vi "Sequence.BuildWaveform.vi"(9 "Rows":cluster{"Start Index":i32, "Length":i32}={"Start Index"=0, "Length"=-1}, 10 "Steps":string[][](array[string]), 11 "Duration":string[](array[string])) -> (1 "Offset":dbl, 2 "Selected":waveform(dbl)[](array[waveform]), 3 "Full":waveform(dbl)[](array[waveform]))   [LabVIEW 2013, in "Simple Sequence Tools - Shared.lvlib"]
uses:
  Simple Sequence Tools - Shared.lvlib
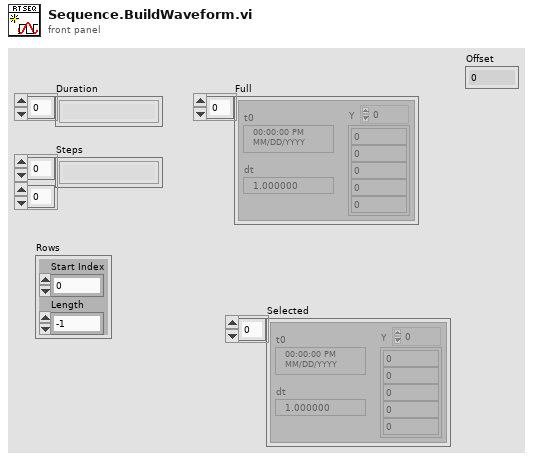
[diagram p1: front panel]
types:
  T1 = typedef "Simple Sequence Tools - Shared.lvlib/Step.Types.ctl" = enum8{"Step", "iStep", "Ramp", "Unchanged", "Unknown", "Sine", "LogSine", "LinearSine", "ForcedRamp", "SquareWave"}
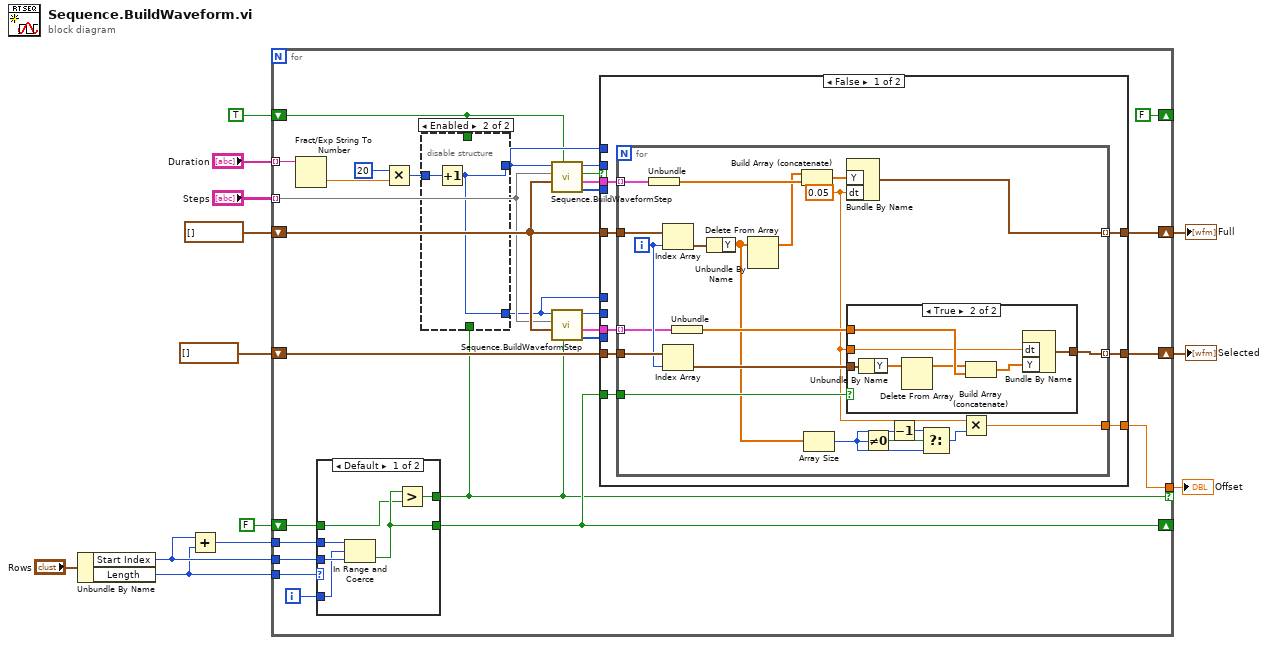
[diagram p0: block diagram]
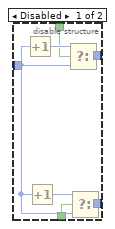
[diagram p2: hidden frame]
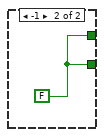
[diagram p3: hidden frame]
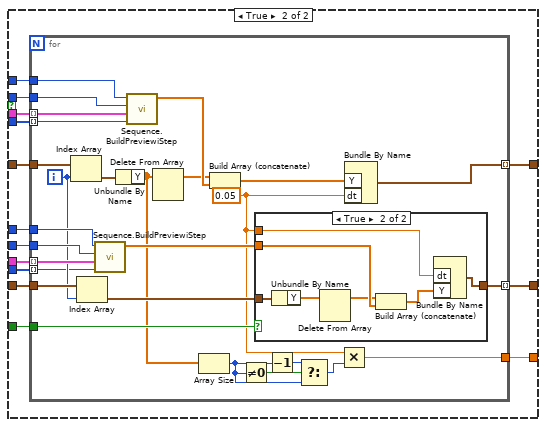
[diagram p5: hidden frame]
diagram:
  n1 = Unbundle By Name("Rows") -> ("Start Index"=w7:i32, "Length"=w6:i32)
  n2 = Add(x=w7, y=w6) -> (x+y=w5:i32)
  n3 = for {
    tunnel: "Steps" -> [w23] mode=indexing
    tunnel: "Duration" -> [w41] mode=indexing
    shift-right: [FALSE] -> _
    shift-left: TRUE -> [w15]
    shift-right: [w34] -> w9
    shift-left: waveform(dbl)[] [] -> [w24]
    tunnel: w6 -> [w33]
    tunnel: w7 -> [w32]
    tunnel: w5 -> [w31]
    shift-right: [w27] -> w3
    shift-left: waveform(dbl)[] [] -> [w28]
    shift-right: [w25] -> _
    shift-left: FALSE -> [w26]
    tunnel: [w18] -> w1 if=w14
    i -> [w30]
    n4 = Fract/Exp String To Number(string=w41) -> (number=w36:dbl)  [unwired: 3 in, 1 out]
    n5 = case shown="Default" w33 {
      tunnel: w32 -> [w56 _]
      tunnel: w31 -> [w55 _]
      tunnel: w30 -> [w54 _]
      tunnel: [w53 w57] -> w25
      tunnel: w26 -> [w52 _]
      tunnel: [w51 w57] -> w14
      frame Default {
        n6 = In Range and Coerce(upper limit=w55, x=w54, lower limit=w56) -> (In Range?=w53:bool)  [unwired: 1 out]
        n7 = Greater?(x=w53, y=w52) -> (0:w51:bool)
      }
      frame -1 {
        w57 = FALSE
      }
    }
    n8 = Multiply(x=u64 20, y=w36) -> (x*y=w22:u64)
    n9 = disable-structure shown="Enabled" {
      disable-tunnel: [w47 w49] -> w35
      disable-tunnel: w22 -> [w45 w50]
      disable-tunnel: [w44 w49] -> w20
      disable-tunnel: w15 -> [w43 _]
      disable-tunnel: w14 -> [w42 _]
      frame Disabled {
        n10 = Increment(x=w45) -> (x+1=w48:u64)
        n11 = Increment(x=w45) -> (x+1=w46:u64)
        n12 = Select(t=w48, s=w43, f=w45) -> (s? t:f=w47:u64)
        n13 = Select(t=w46, s=w42, f=w45) -> (s? t:f=w44:u64)
      }
      frame Enabled {
        n14 = Increment(x=w50) -> (x+1=w49:u64)
      }
    }
    n15 = call "Sequence.BuildWaveformStep.vi"("FirstIteration"=w15, "Current Waveform"=w24, "Steps"=w23, "DataPoints"=w35) -> ("Step Type"=w17:T1[], "IO Points"=w38:cluster{"Ramp Pattern":dbl[]}[], "iStep"=w40:bool, "iStep Size"=w39:i32)  [unwired: 4 in]
    n16 = call "Sequence.BuildWaveformStep.vi"("FirstIteration"=w14, "Current Waveform"=w24, "Steps"=w23, "DataPoints"=w20) -> ("Step Type"=w16:T1[], "IO Points"=w19:cluster{"Ramp Pattern":dbl[]}[], "iStep Size"=w21:i32)  [unwired: 4 in, 1 out]
    n17 = case shown="False" w40 {
      tunnel: w39 -> [_ w107]
      tunnel: w38 -> [w65 w108]
      tunnel: w35 -> [_ w106]
      tunnel: [w64 w105] -> w34
      tunnel: w24 -> [w63 w104]
      tunnel: w28 -> [w62 w103]
      tunnel: w25 -> [w61 w102]
      tunnel: [w60 w101] -> w27
      tunnel: w21 -> [_ w100]
      tunnel: w20 -> [_ w99]
      tunnel: w19 -> [w59 w98]
      tunnel: [w58 w97] -> w18
      tunnel: w17 -> [_ w96]
      tunnel: w16 -> [_ w95]
      frame False {
        n18 = for {
          tunnel: w65 -> [w86] mode=indexing
          tunnel: [w85] -> w64 mode=indexing
          tunnel: w63 -> [w83]
          tunnel: w62 -> [w81]
          tunnel: w61 -> [w78]
          tunnel: [w79] -> w60 mode=indexing
          tunnel: w59 -> [w75] mode=indexing
          tunnel: [w68] -> w58
          i -> [w80]
          w69 = 0.05 ("dt")
          n19 = Unbundle(w86) -> ("Ramp Pattern"=w76:dbl[])
          n20 = Index Array(array=w83, index=w80) -> (element=w82:waveform(dbl))
          n21 = Index Array(array=w81, index=w80) -> (element=w77:waveform(dbl))
          n22 = Unbundle(w75) -> ("Ramp Pattern"=w74:dbl[])
          n23 = Unbundle By Name(w82) -> ("Y"=w66:dbl[])
          n24 = Delete From Array(array=w66) -> (array with subset deleted=w67:dbl[])  [unwired: 2 in, 1 out]
          n25 = Build Array (concatenate)(w67, w76) -> (w84:dbl[])
          n26 = Array Size(array=w66) -> (size(s)=w70:i32)
          n27 = Bundle By Name("Y"=w84, "dt"=w69) -> (w85:waveform(dbl))  [unwired: 1 in]
          n28 = case shown="True" w78 {
            tunnel: w69 -> [_ w88]
            tunnel: [w87 w93] -> w79
            tunnel: w77 -> [w87 w92]
            tunnel: w74 -> [_ w91]
            frame False {
            }
            frame True {
              n29 = Unbundle By Name(w92) -> ("Y"=w90:dbl[])
              n30 = Delete From Array(array=w90) -> (array with subset deleted=w89:dbl[])  [unwired: 2 in, 1 out]
              n31 = Build Array (concatenate)(w89, w91) -> (w94:dbl[])
              n32 = Bundle By Name("dt"=w88, "Y"=w94) -> (w93:waveform(dbl))  [unwired: 1 in]
            }
          }
          n33 = Not Equal To 0?(x=w70) -> (x != 0?=w71:bool)
          n34 = Decrement(x=w70) -> (x-1=w73:i32)
          n35 = Select(t=w73, s=w71, f=w70) -> (s? t:f=w72:i32)
          n36 = Multiply(x=w69, y=w72) -> (x*y=w68:dbl)
        }
      }
      frame True {
        n37 = for {
          tunnel: w108 -> [w134] mode=indexing
          tunnel: w107 -> [w135]
          tunnel: w106 -> [w133]
          tunnel: [w132] -> w105 mode=indexing
          tunnel: w104 -> [w130]
          tunnel: w103 -> [w127]
          tunnel: w102 -> [w126]
          tunnel: [w125] -> w101 mode=indexing
          tunnel: w100 -> [w123]
          tunnel: w99 -> [w122]
          tunnel: w98 -> [w121] mode=indexing
          tunnel: [w117] -> w97
          tunnel: w96 -> [w112] mode=indexing
          tunnel: w95 -> [w111] mode=indexing
          i -> [w119]
          w118 = 0.05 ("dt")
          n38 = Index Array(array=w130, index=w119) -> (element=w129:waveform(dbl))
          n39 = Index Array(array=w127, index=w119) -> (element=w128:waveform(dbl))
          n40 = call "Sequence.BuildPreviewiStep.vi"("Step"=w111, "Step IO"=w121, "iStep Iterations"=w123, "Step Duration"=w122) -> ("Ramp Pattern"=w120:dbl[])  [unwired: 7 in]
          n41 = Unbundle By Name(w129) -> ("Y"=w109:dbl[])
          n42 = call "Sequence.BuildPreviewiStep.vi"("Step"=w112, "Step IO"=w134, "iStep Iterations"=w135, "Step Duration"=w133) -> ("Ramp Pattern"=w124:dbl[])  [unwired: 7 in]
          n43 = Delete From Array(array=w109) -> (array with subset deleted=w110:dbl[])  [unwired: 2 in, 1 out]
          n44 = Array Size(array=w109) -> (size(s)=w114:i32)
          n45 = Build Array (concatenate)(w110, w124) -> (w131:dbl[])
          n46 = Not Equal To 0?(x=w114) -> (x != 0?=w116:bool)
          n47 = case shown="True" w126 {
            tunnel: w120 -> [_ w143]
            tunnel: w118 -> [_ w139]
            tunnel: [w136 w141] -> w125
            tunnel: w128 -> [w136 w140]
            frame False {
            }
            frame True {
              n48 = Unbundle By Name(w140) -> ("Y"=w138:dbl[])
              n49 = Delete From Array(array=w138) -> (array with subset deleted=w137:dbl[])  [unwired: 2 in, 1 out]
              n50 = Build Array (concatenate)(w137, w143) -> (w142:dbl[])
              n51 = Bundle By Name("dt"=w139, "Y"=w142) -> (w141:waveform(dbl))  [unwired: 1 in]
            }
          }
          n52 = Decrement(x=w114) -> (x-1=w113:i32)
          n53 = Select(t=w113, s=w116, f=w114) -> (s? t:f=w115:i32)
          n54 = Multiply(x=w118, y=w115) -> (x*y=w117:dbl)
          n55 = Bundle By Name("Y"=w131, "dt"=w118) -> (w132:waveform(dbl))  [unwired: 1 in]
        }
      }
    }
  }
  "Full" <- w9
  "Selected" <- w3
  "Offset" <- w1
